vi "led_cntl_arduino.vi"() -> ()   [LabVIEW 2017]
uses:
  <vilib>/Instr/_visa.llb/VISA Configure Serial Port (Instr).vi
panel:
  in  "串口号":refnum<visa-resource-name>
  out "LED":bool
  in  "Turn On Button":bool
  in  "Turn Off Button":bool
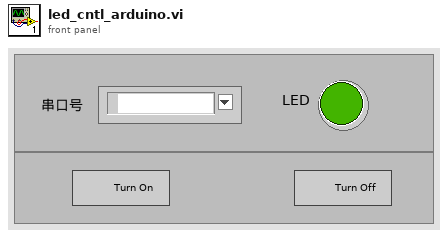
[diagram p1: front panel]
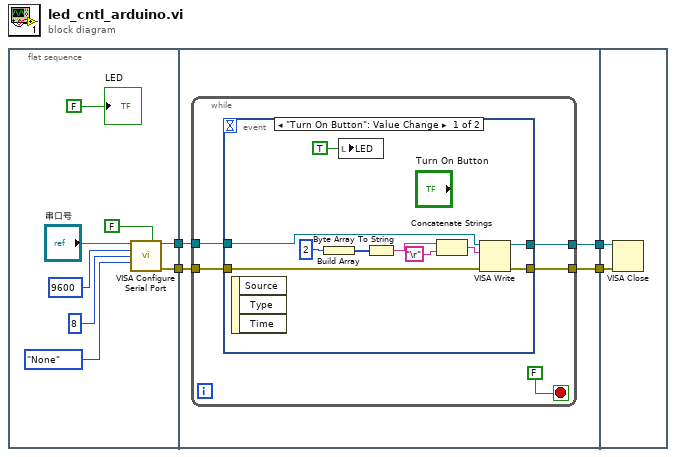
[diagram p0: block diagram]
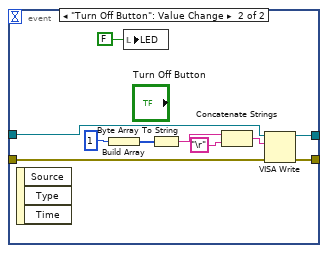
[diagram p2: hidden frame]
diagram:
  n1 = flat-sequence {
    tunnel: [w8] -> w4
    tunnel: [w7] -> w3
    tunnel: w4 -> [w16]
    tunnel: w3 -> [w15]
    tunnel: [w14] -> w2
    tunnel: [w13] -> w1
    tunnel: w2 -> [w43]
    tunnel: w1 -> [w42]
    frame #0 {
      n2 = call-poly "VISA Configure Serial Port"("VISA resource name"="串口号", "Enable Termination\nChar (T)"=FALSE, "baud rate (9600)"=9600, "data bits (8)"=8, "parity (0:none)"=enum16{"None", "Odd", "Even", "Mark", "Space"}."None") -> ("VISA resource name out"=w8:refnum<visa-resource-name>, "error out"=w7:errorcluster)  [unwired: 9 in]
      "LED" <- FALSE
    }
    frame #1 {
      n3 = while {
        tunnel: w16 -> [w19]
        tunnel: w15 -> [w21]
        tunnel: [w20] -> w14
        tunnel: [w18] -> w13
        stop <- FALSE stop-if-true
        n4 = event shown="[0] \"Turn On Button\": Value Change" {
          selector: _ -> [_ _]
          dyn-events: _ -> [_ _]
          timeout: _ -> [_ _]
          tunnel: w21 -> [w31 w34]
          tunnel: [w30 w35] -> w20
          tunnel: w19 -> [w29 w33]
          tunnel: [w28 w36] -> w18
          event "Turn On Button": Value Change {
            n5 = event-data() -> ()  [unwired: 1 in, 3 out]
            n6 = Build Array(2) -> (w24:i32[])
            n7 = local write "LED"(TRUE) -> ()
            n8 = Byte Array To String(unsigned byte array=w24) -> (string=w26:string)
            n9 = Concatenate Strings(w26, "\r") -> (w23:string)
            n10 = VISA Write(VISA resource name=w29, write buffer=w23, error in (no error)=w31) -> (VISA resource name out=w28:refnum<visa-resource-name>, error out=w30:errorcluster)  [unwired: 1 out]
          }
          event "Turn Off Button": Value Change {
            n11 = event-data() -> ()  [unwired: 1 in, 3 out]
            n12 = Build Array(1) -> (w38:i32[])
            n13 = local write "LED"(FALSE) -> ()
            n14 = Byte Array To String(unsigned byte array=w38) -> (string=w40:string)
            n15 = Concatenate Strings(w40, "\r") -> (w37:string)
            n16 = VISA Write(VISA resource name=w33, write buffer=w37, error in (no error)=w34) -> (VISA resource name out=w36:refnum<visa-resource-name>, error out=w35:errorcluster)  [unwired: 1 out]
          }
        }
      }
    }
    frame #2 {
      n17 = VISA Close(VISA resource name=w42, error in (no error)=w43) -> ()  [unwired: 1 out]
    }
  }
